vi "App2_Light_Leds.vi"() -> ()   [LabVIEW 2022 SP3]
uses:
  <vilib>/DAQmx/read.llb/DAQmx Read (Analog DBL 1Chan 1Samp).vi
  <vilib>/DAQmx/write.llb/DAQmx Write (Digital 1D Bool NChan 1Samp 1Line).vi
  <vilib>/DAQmx/miscellaneous.llb/DAQmx Fill In Error Info.vi
panel:
  out "Led Level Light":bool[](array[boolean])
  out "Waveform Chart":dbl(graph)
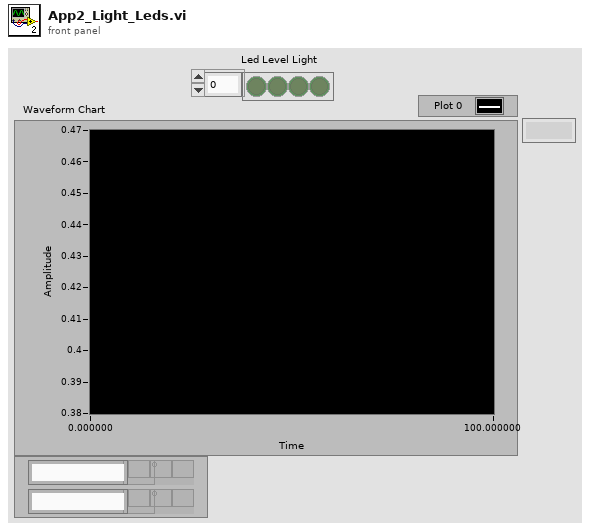
[diagram p1: front panel]
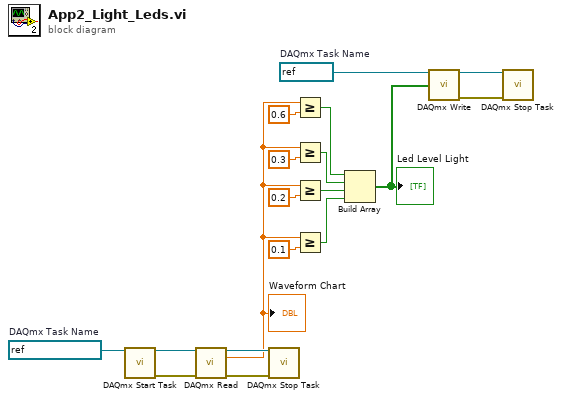
[diagram p0: block diagram]
diagram:
  w2 = refnum<k21> "LEDS"  # DAQmx Task Name
  w14 = refnum<k21> "Light Sensor"  # DAQmx Task Name
  n1 = call <vilib>:"DAQmx Start Task.vi"("task/channels in"=w14) -> ("task out"=w16:refnum<k21>, "error out"=w18:errorcluster)  [unwired: 13 in]
  n2 = call-poly <vilib>:"DAQmx Read.vi"("task/channels in"=w16, "error in"=w18) -> ("task out"=w15:refnum<k21>, "data"=w9:dbl, "error out"=w17:errorcluster)  [unwired: 11 in]
  "Waveform Chart" <- w9
  n3 = call <vilib>:"DAQmx Stop Task.vi"("task/channels in"=w15, "error in"=w17) -> ()  [unwired: 12 in, 2 out]
  n4 = Greater Or Equal?(x=w9, y=0.6) -> (x >= y?=w8:bool)
  n5 = Greater Or Equal?(x=w9, y=0.3) -> (x >= y?=w7:bool)
  n6 = Greater Or Equal?(x=w9, y=0.2) -> (x >= y?=w6:bool)
  n7 = Greater Or Equal?(x=w9, y=0.1) -> (x >= y?=w5:bool)
  n8 = Build Array(w8, w7, w6, w5) -> (w1:bool[])
  "Led Level Light" <- w1
  n9 = call-poly <vilib>:"DAQmx Write.vi"("task/channels in"=w2, "data"=w1) -> ("task out"=w3:refnum<k21>, "error out"=w4:errorcluster)  [unwired: 11 in, 1 out]
  n10 = call <vilib>:"DAQmx Stop Task.vi"("task/channels in"=w3, "error in"=w4) -> ()  [unwired: 12 in, 2 out]
